vi "Scalar Vector Matrix Info.vi"(11 "octave sizes":i32[](array[numeric])) -> (0 "is >2d matrix?":bool, 1 "is matrix?":bool, 2 "is vector?":bool, 3 "is scalar?":bool, 4 "row vector?":bool, 5 "vector length":i32=-1)   [LabVIEW 2013, in "GOLPI library.lvlib"]
doc: "Returns if object determined by sizes specified on input is scalar, vector or matrix. If vector, returns if is row vector and returns length of the vector. Sizes are in GNU Octave metrics (no elements withzero indexes). Mathematically, x=[1] is scalar and also is vector and also is matrix, however this vi returns only one possibility."
uses:
  GOLPI library.lvlib
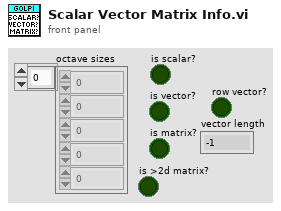
[diagram p1: front panel]
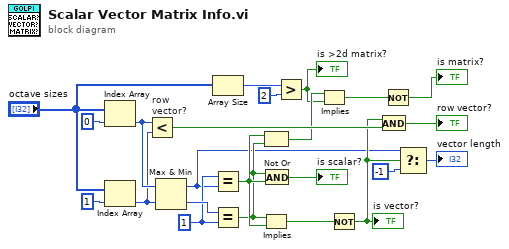
[diagram p0: block diagram]
diagram:
  w18 = 1 ("y")
  n1 = Index Array(array="octave sizes", index=0) -> (element=w21:i32)
  n2 = Index Array(array="octave sizes", index=1) -> (element=w20:i32)
  n3 = Less? "row\nvector?"(x=w21, y=w20) -> (x < y?=w10:bool)
  n4 = Max & Min(x=w21, y=w20) -> (max(x,y)=w3:i32, min(x,y)=w19:i32)
  n5 = Array Size(array="octave sizes") -> (size(s)=w11:i32)
  n6 = Equal?(x=w18, y=w3) -> (x = y?=w14:bool)
  n7 = Equal?(x=w19, y=w18) -> (x = y?=w12:bool)
  n8 = Not Or(1:w12, 2:w14) -> (0:w7:bool)
  n9 = Implies(1:w14, 2:w12) -> (0:w13:bool)
  n10 = And(x=w12, y=w14) -> (x .and. y?=→"is scalar?":bool)
  n11 = Greater?(x=w11, y=2) -> (0:w6:bool)
  "is >2d matrix?" <- w6
  n12 = Implies(1:w6, 2:w7) -> (0:w8:bool)
  n13 = Not(x=w13) -> (.not. x?=w4:bool)
  "is vector?" <- w4
  n14 = And(x=w4, y=w10) -> (x .and. y?=→"row vector?":bool)
  n15 = Not(x=w8) -> (.not. x?=→"is matrix?":bool)
  n16 = Select(t=w3, s=w4, f=-1) -> (s? t:f=→"vector length":i32)
